vi "Full Join.vi"() -> ()   [LabVIEW 2020]
uses:
  a75eeadb-a20a-426b-b48b-c9c06ab4b909.vi
  965599a9-35c5-4084-8906-0a043779e57e.vi
panel:
  out "array with duplicates removed":string[][](array[string])
  in  "Array 2":string[][](array[string])
  in  "Array":string[][](array[string])
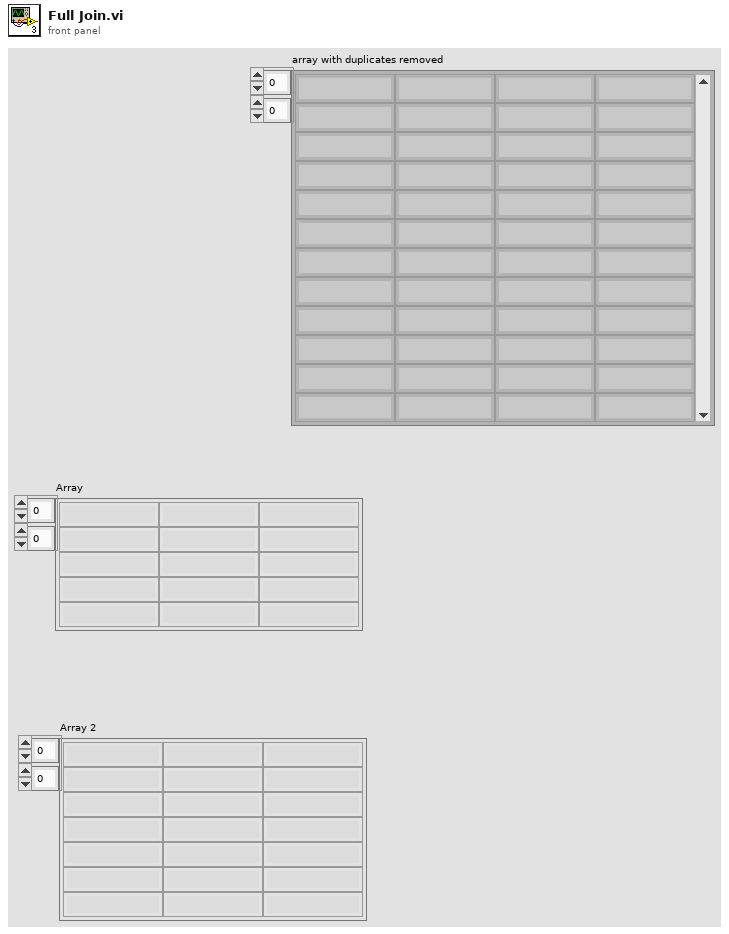
[diagram p1: front panel]
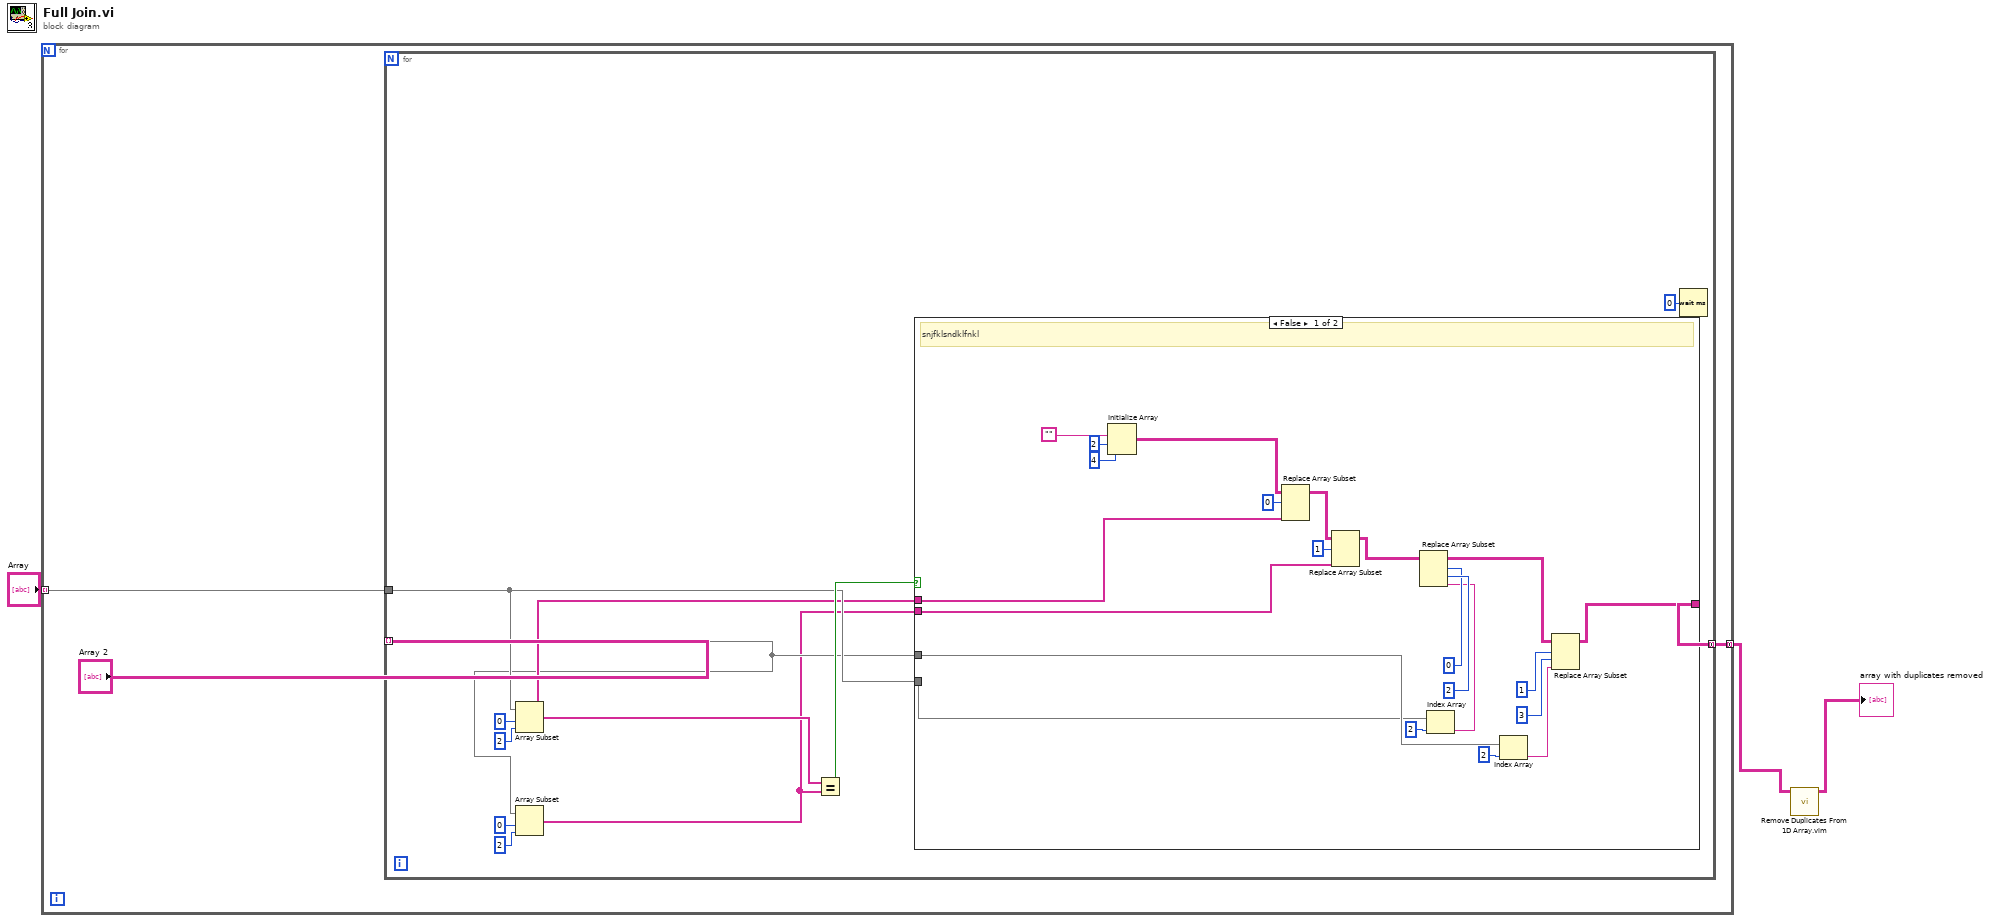
[diagram p0: block diagram]
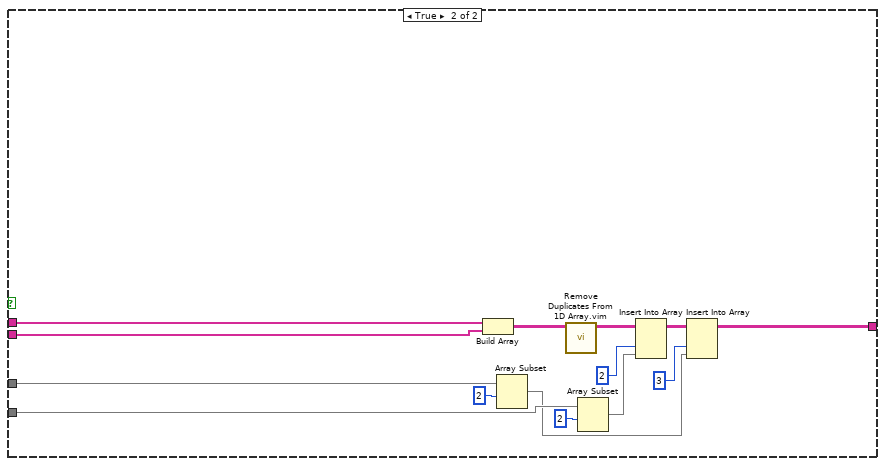
[diagram p2: hidden frame]
diagram:
  n1 = for {
    tunnel: "Array" -> [w5] mode=indexing
    tunnel: [w6] -> w2 mode=concatenating
    n2 = for {
      tunnel: "Array 2" -> [w9] mode=indexing
      tunnel: w5 -> [w11]
      tunnel: [w16] -> w6 mode=concatenating
      n3 = Array Subset(array=w11, index=0, length=2) -> (w10:string[])
      n4 = Array Subset(array=w9, index=0, length=2) -> (w8:string[])
      n5 = Equal?(x=w10, y=w8) -> (x = y?=w17:bool)
      n6 = case shown="False" w17 {
        tunnel: [w18 w42] -> w16
        tunnel: w11 -> [w36 w49]
        tunnel: w9 -> [w37 w46]
        tunnel: w10 -> [w23 w53]
        tunnel: w8 -> [w22 w52]
        frame False {
          # "snjfklsndklfnkl"
          n7 = Initialize Array("", 2 ("dimension size"), 4 ("dimension size")) -> (w25:string[][])
          n8 = Replace Array Subset(array=w25, new element=w23, index (row)=0) -> (w24:string[][])  [unwired: 1 in]
          n9 = Replace Array Subset(array=w24, new element=w22, index (row)=1) -> (w19:string[][])  [unwired: 1 in]
          n10 = Index Array(array=w36, index=2) -> (element=w31:string)
          n11 = Replace Array Subset(array=w19, new element=w31, index (row)=0 ("disabled index (row)"), index (col)=2 ("index (row)")) -> (w34:string[][])
          n12 = Index Array(array=w37, index=2) -> (element=w38:string)
          n13 = Replace Array Subset(array=w34, new element=w38, index (row)=1 ("disabled index (row)"), index (col)=3 ("index (row)")) -> (w18:string[][])
        }
        frame True {
          n14 = Build Array(w53, w52) -> (w51:string[][])
          n15 = Array Subset(array=w46, index=2) -> (w43:string[])  [unwired: 1 in]
          n16 = call "Remove Duplicates From 1D Array.vim"("array"=w51) -> ("array with duplicates removed"=w50:string[][])  [unwired: 10 in]
          n17 = Array Subset(array=w49, index=2) -> (w48:string[])  [unwired: 1 in]
          n18 = Insert Into Array(array=w50, index (col)=2 ("index (row)"), new element=w48) -> (w44:string[][])  [unwired: 1 in]
          n19 = Insert Into Array(array=w44, index (col)=3 ("index (row)"), new element=w43) -> (w42:string[][])  [unwired: 1 in]
        }
      }
      n20 = Wait (ms)(milliseconds to wait=u32 0) -> ()  [unwired: 1 out]
    }
  }
  n21 = call "Remove Duplicates From 1D Array.vim"("array"=w2) -> ("array with duplicates removed"=→"array with duplicates removed":string[][])  [unwired: 10 in]
